vi "Log Values Example.vi"() -> ()   [LabVIEW 2017, in "Logger Examples.lvlib"]
uses:
  Logger Examples.lvlib
  Source/Composed Log/Types/Log Level.ctl
  Source/String Formats/String Expression Format/String Expression Format.lvclass/String Expression Format.ctl
  Source/Composed Log/LoggerReference/LoggerReference.lvclass/LoggerReference.ctl
  cb6cc8f4-355e-4f60-beee-1dac019a5190.vi
  d053d638-c5ca-4061-b75c-930c5d54a4a0.vi
  a4aecb2a-c8ab-40e1-948d-3fbd1094d214.vi
  d9747495-8d6c-4d86-9b58-ec7b36ea6678.vi
  13ff8fb6-9e5d-4405-b0df-27c05d5aea20.vi
  9f234408-1270-49d7-b342-8c2f3c962d83.vi
  150d9d2d-db35-4e36-bc8e-367fbd223884.vi
  57f424a8-0347-4995-a908-3cdd2378fbfa.vi
  261ea4dc-86e2-4e22-a46e-fc1e124681f7.vi
  Source/String Formats/String Expression Format/Run Formatter.vi
  Source/Composed Log/LoggerReference/Return Aggregate Queues.vi
  Source/Composed Log/LoggerReference/Add Aggregate Log.vi
  cb6cc8f4-355e-4f60-beee-1dac019a5190.vi/f0589759-63da-4caa-be49-6820fd9972fe.vi
  a4aecb2a-c8ab-40e1-948d-3fbd1094d214.vi/99aec1de-331a-4b74-ab39-78b7e0dff1d5.vi
  Source/Composed Log/LoggerReference/Log Event.vi
  d9747495-8d6c-4d86-9b58-ec7b36ea6678.vi/3ca36584-379f-4a74-bf28-aba9d29f22e9.vi
  13ff8fb6-9e5d-4405-b0df-27c05d5aea20.vi/c7f29d47-fbe0-4db9-bfd7-545af0b20a9e.vi
  9f234408-1270-49d7-b342-8c2f3c962d83.vi/642c3834-3724-42ee-9e99-4ee14d18eccc.vi
  150d9d2d-db35-4e36-bc8e-367fbd223884.vi/46f88a2b-4662-4e92-a40f-b9227fc573ce.vi
  57f424a8-0347-4995-a908-3cdd2378fbfa.vi/5a08e50a-33f3-4eb7-9d66-0f6109bda26b.vi
  Source/Composed Log/LoggerReference/Get Formatter.vi
  261ea4dc-86e2-4e22-a46e-fc1e124681f7.vi/f7ba94e1-af1b-40a6-9210-a60f7f8d15a0.vi
  <vilib>/dlg_ctls.llb/Space Constant.vi
  Source/Composed Log/LoggerReference/Send Add Sink.vi
  Source/Composed Log/LoggerReference/Log.vi
  Source/Composed Log/LoggerReference/Remove Stale Logs.vi
  Source/String Formats/String Expression Format/String Expression Format.lvclass
  C:/CS/Internal/LabVIEW/Logger/Source/IStringFormat/IStringFormat.lvclass
  Source/String Control Sink/String Control Sink.lvclass
  C:/CS/Internal/LabVIEW/Logger/Source/Composed Log/Log Sink/Log Sink.lvclass
  Source/Composed Log/Application Logger/Launch Worker Loop.vi
  Source/Composed Log/LoggerReference/Initialize Logger Instance.vi
  Source/Composed Log/LoggerReference/Format Variant.vi
  Source/Composed Log/LoggerReference/LoggerReference.lvclass
  Source/Composed Log/IErrorFormat/IErrorFormat.lvclass
  Source/Composed Log/Log Sink/Log Sink.lvclass
  GenericSerializable/GenericSerializable.lvclass
  Source/Composed Log/Composed Log.lvlib
panel:
  out "Event Log":string
  # "Run the VI, then view the block diagram notes for details on formatting various data types."
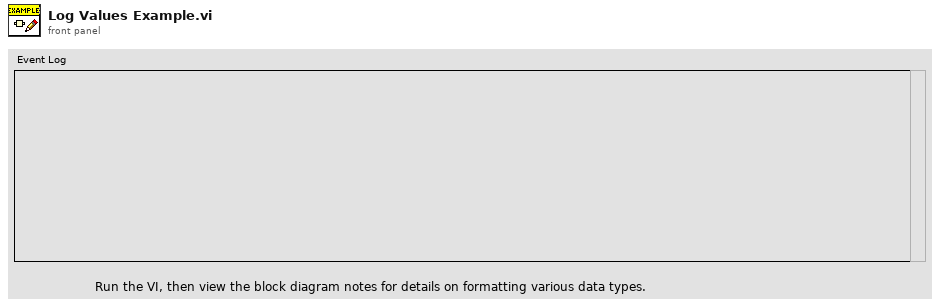
[diagram p1: front panel]
types:
  T1 = typedef "Composed Log.lvlib/Log Level.ctl" = enum16{"Debug", "Info", "Warning", "Error", "Critical"}
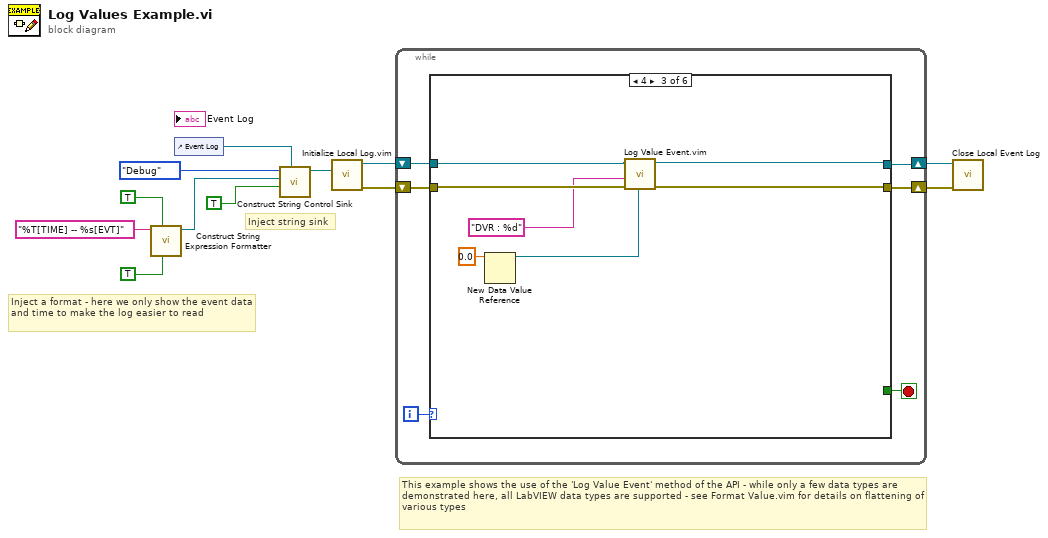
[diagram p0: block diagram]
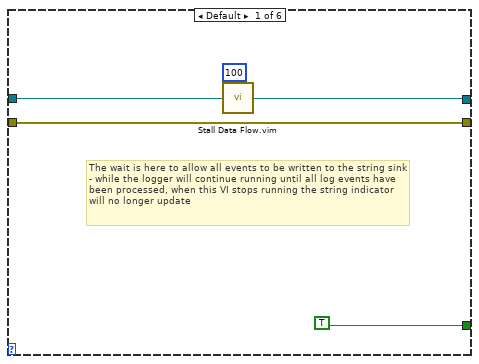
[diagram p2: hidden frame]
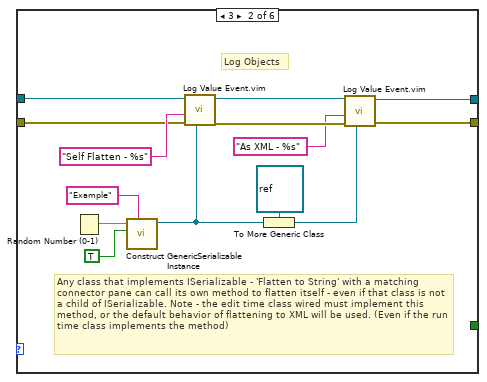
[diagram p3: hidden frame]
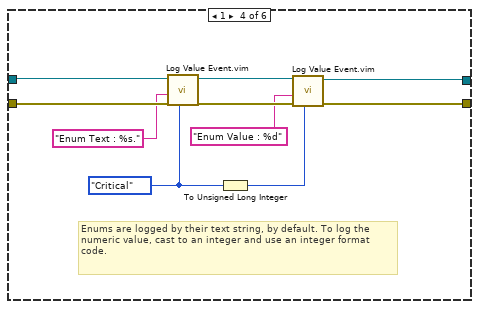
[diagram p4: hidden frame]
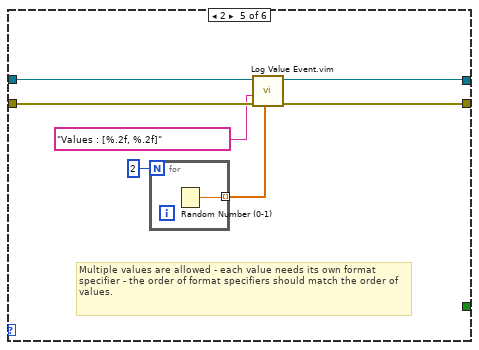
[diagram p5: hidden frame]
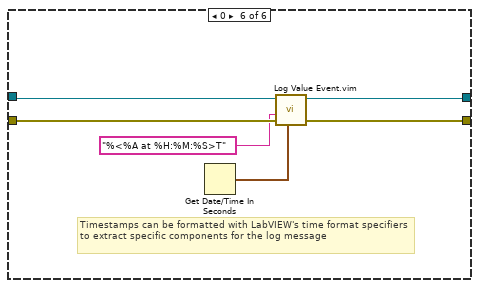
[diagram p6: hidden frame]
diagram:
  # "This example shows the use of the 'Log Value Event' method of the API - while only a few data types are demonstrated here, all LabVIEW data types are supported - see Format Value.vim for details on flattening of various types"
  # "Inject string sink"
  # "Inject a format - here we only show the event data and time to make the log easier to read"
  n1 = call "Construct String Expression Formatter.vi"("Remove LineFeeds?(F)"=TRUE, "Append EOL?"=TRUE, "Format Specifier"="%T[TIME] -- %s[EVT]") -> ("String Expression Format out"=w9:refnum<class "String Expression Format.lvclass">)  [unwired: 7 in, 1 out]
  n2 = control-ref of="Event Log"() -> (w11:refnum<vi>)
  n3 = call "Construct String Control Sink.vi"("Str Refnum"=w11, "AutoScroll?(F)"=TRUE, "LogFormat"=w9, "LogLevel"=Log_Level."Debug") -> ("String Control Sink out"=w1:refnum<class "String Control Sink.lvclass">)  [unwired: 7 in]
  n4 = call "Initialize Local Log.vim"("Startup Sink(s)"=w1) -> ("error out"=w5:errorcluster, "Log Instance Reference"=w4:refnum<class "LoggerReference.lvclass">)  [unwired: 8 in, 1 out]
  n5 = while {
    shift-right: [w15] -> w2
    shift-left: w5 -> [w18]
    shift-right: [w16] -> w3
    shift-left: w4 -> [w17]
    i -> [w14]
    stop <- w13 stop-if-true
    n6 = case shown="4" w14 {
      tunnel: w18 -> [w23 w26 w42 w51 w57 w65]
      tunnel: w17 -> [w20 w27 w43 w52 w58 w66]
      tunnel: [w19 w31 w38 w53 w59 w68] -> w16
      tunnel: [w23 w30 w39 w54 w60 w67] -> w15
      tunnel: [TRUE _ _ _ _ _] -> w13
      frame Default {
        # "The wait is here to allow all events to be written to the string sink - while the logger will continue running until all log events have been processed, when this VI stops running the string indicator will no longer update"
        n7 = call "Stall Data Flow.vim"("value in"=w20, "milliseconds to wait"=u32 100) -> ("value out"=w19:refnum<class "LoggerReference.lvclass">)  [unwired: 1 out]
      }
      frame 3 {
        # "Log Objects"
        # "Any class that implements ISerializable - 'Flatten to String' with a matching connector pane can call its own method to flatten itself - even if that class is not a child of ISerializable. Note - the edit time class wired must implement this method, or the default behavior of flattening to XML will be used. (Even if the run time class implements the method)"
        n8 = Random Number (0-1)() -> (number: 0 to 1=w35:dbl)
        n9 = call "Construct GenericSerializable Instance.vi"("InstanceID"="Example", "Boolean Data"=TRUE, "Numeric Data"=w35) -> ("GenericSerializable out"=w25:refnum<class "GenericSerializable.lvclass">)  [unwired: 8 in]
        n10 = call "Log Value Event.vim"("Value(s)"=w25, "error in (no error)"=w26, "Log Message Format String"="Self Flatten - %s" ("Log Message"), "LoggerReference in"=w27) -> ("error out"=w32:errorcluster, "LoggerReference out"=w33:refnum<class "LoggerReference.lvclass">)  [unwired: 6 in]
        n11 = To More Generic Class(target class=refnum<class> refnum ("LabVIEW Object"), reference=w25) -> (generic class reference=w24:refnum<class>)
        n12 = call "Log Value Event.vim"("Value(s)"=w24, "error in (no error)"=w32, "Log Message Format String"="As XML - %s" ("Log Message"), "LoggerReference in"=w33) -> ("error out"=w30:errorcluster, "LoggerReference out"=w31:refnum<class "LoggerReference.lvclass">)  [unwired: 6 in]
      }
      frame 4 {
        n13 = New Data Value Reference(data value=0.0) -> (data value reference=w41:refnum<data-value>)  [unwired: 1 in, 1 out]
        n14 = call "Log Value Event.vim"("Value(s)"=w41, "error in (no error)"=w42, "Log Message Format String"="DVR : %d", "LoggerReference in"=w43) -> ("error out"=w39:errorcluster, "LoggerReference out"=w38:refnum<class "LoggerReference.lvclass">)  [unwired: 6 in]
      }
      frame 1 {
        w46 = Log_Level."Critical" ("Event Level")
        # "Enums are logged by their text string, by default. To log the numeric value, cast to an integer and use an integer format code."
        n15 = call "Log Value Event.vim"("Value(s)"=w46, "error in (no error)"=w51, "Log Message Format String"="Enum Text : %s." ("Log Message"), "LoggerReference in"=w52) -> ("error out"=w49:errorcluster, "LoggerReference out"=w50:refnum<class "LoggerReference.lvclass">)  [unwired: 6 in]
        n16 = To Unsigned Long Integer(number=w46) -> (unsigned 32bit integer=w45:u32)
        n17 = call "Log Value Event.vim"("Value(s)"=w45, "error in (no error)"=w49, "Log Message Format String"="Enum Value : %d" ("Log Message"), "LoggerReference in"=w50) -> ("error out"=w54:errorcluster, "LoggerReference out"=w53:refnum<class "LoggerReference.lvclass">)  [unwired: 6 in]
      }
      frame 2 {
        # "Multiple values are allowed - each value needs its own format specifier - the order of format specifiers should match the order of values."
        n18 = for {
          N: 2 -> [_]
          tunnel: [w62] -> w55 mode=indexing
          n19 = Random Number (0-1)() -> (number: 0 to 1=w62:dbl)
        }
        n20 = call "Log Value Event.vim"("Value(s)"=w55, "error in (no error)"=w57, "Log Message Format String"="Values : [%.2f, %.2f]" ("Log Message"), "LoggerReference in"=w58) -> ("error out"=w60:errorcluster, "LoggerReference out"=w59:refnum<class "LoggerReference.lvclass">)  [unwired: 6 in]
      }
      frame 0 {
        # "Timestamps can be formatted with LabVIEW's time format specifiers to extract specific components for the log message"
        n21 = Get Date/Time In Seconds() -> (seconds since 1Jan1904=w64:timestamp)
        n22 = call "Log Value Event.vim"("Value(s)"=w64, "error in (no error)"=w65, "Log Message Format String"="%<%A at %H:%M:%S>T", "LoggerReference in"=w66) -> ("error out"=w67:errorcluster, "LoggerReference out"=w68:refnum<class "LoggerReference.lvclass">)  [unwired: 6 in]
      }
    }
  }
  n23 = call "Close Local Event Log.vi"("error in (no error)"=w2, "Log Instance"=w3) -> ()  [unwired: 9 in, 1 out]
